vi "XML Build Entity.vi"(0 "Attributes":string[](array[string]), 1 "level":i32, 3 "spaces per level":i32, 5 "Entity Name":string, 7 "Is Array?":bool, 9 "Has Children":bool, 11 "error in (no error)":errorcluster, 12 "Child Entities":string[](array[string])) -> (6 "Entity XML":string, 15 "error out":errorcluster)   [LabVIEW 2016]
doc: "PBrooks - 29 Oct 2018\n\nAdded space to Close Entity? string suffix for compliance to XML spec"
uses:
  <userlib>/_OpenG.lib/array/array.llb/Filter 1D Array (String)__ogtk.vi
  <userlib>/_OpenG.lib/array/array.llb/Empty 1D Array (String)__ogtk.vi
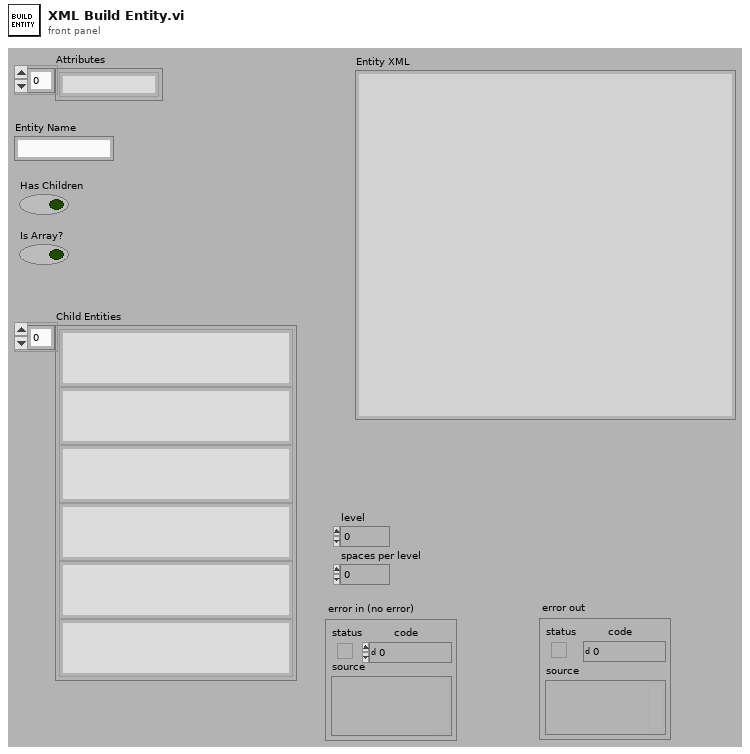
[diagram p1: front panel]
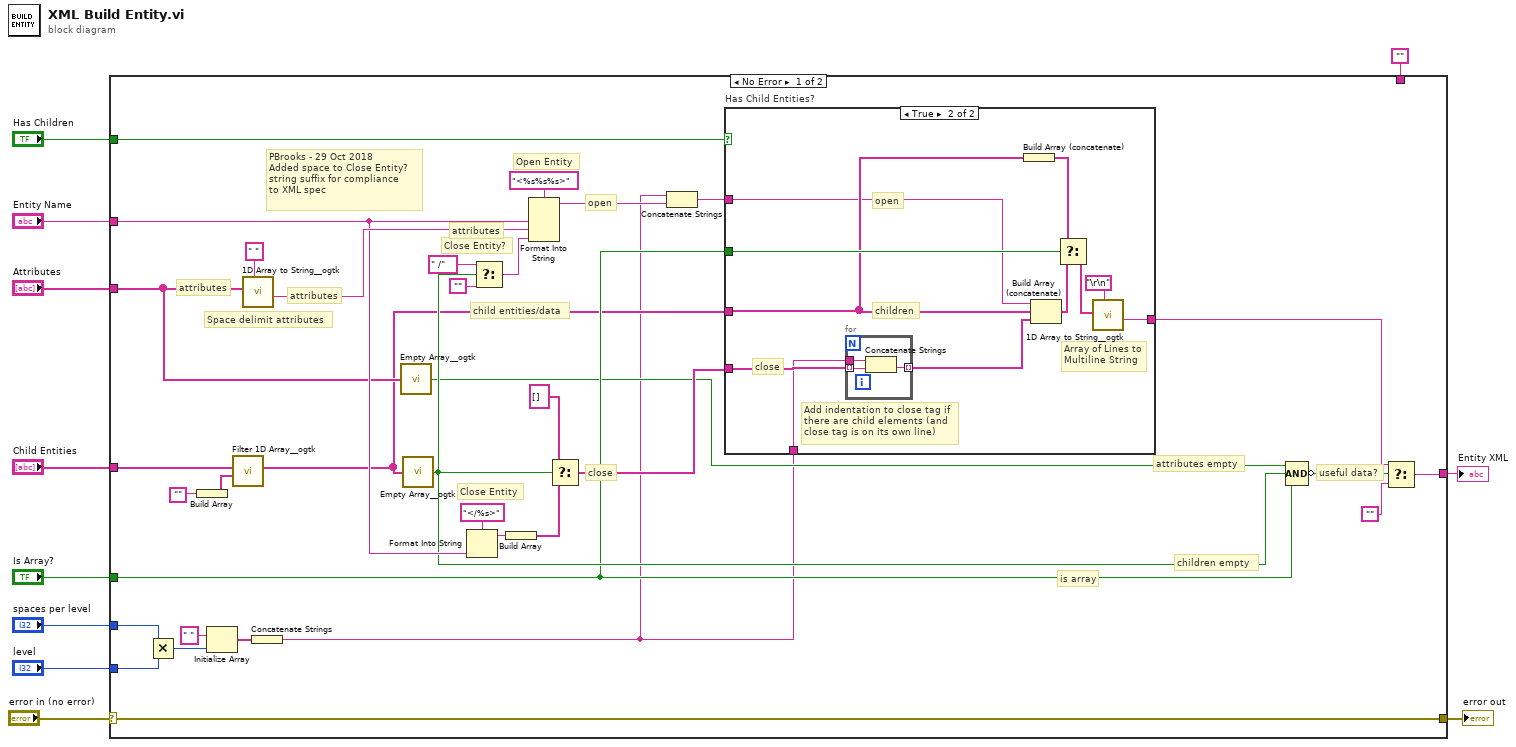
[diagram p0: block diagram]
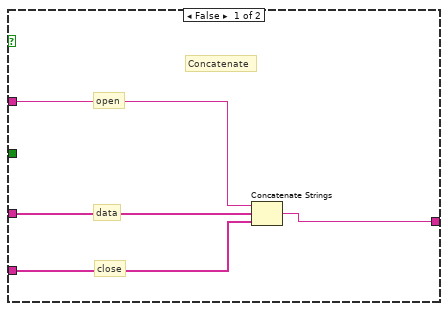
[diagram p2: hidden frame]
diagram:
  n1 = case shown="No Error" "error in (no error)" {
    selector: "error in (no error)" -> [w12 w65]
    tunnel: "Has Children" -> [w45 _]
    tunnel: "Entity Name" -> [w34 _]
    tunnel: "Attributes" -> [w32 _]
    tunnel: "Is Array?" -> [w30 _]
    tunnel: [w26 w64] -> w7
    tunnel: "Child Entities" -> [w23 _]
    tunnel: "spaces per level" -> [w19 _]
    tunnel: "level" -> [w18 _]
    tunnel: [w12 w65] -> w2
    tunnel: "" -> [_ w64]
    frame No Error {
      # "PBrooks - 29 Oct 2018\nAdded space to Close Entity?\nstring suffix for compliance\nto XML spec"
      # "useful data?"
      # "is array"
      # "children empty"
      # "attributes empty"
      # "attributes"
      # "open"
      # "close"
      # "child entities/data"
      # "attributes"
      # "attributes"
      # "Space delimit attributes"
      # "Close Entity?"
      # "Open Entity"
      # "Close Entity"
      n2 = Multiply(x=w19, y=w18) -> (x*y=w17:i32)
      n3 = Build Array("") -> (w21:string[])
      n4 = Initialize Array(" " ("delimiter (Tab)"), w17) -> (w20:string[])
      n5 = call-poly <userlib>:"Filter 1D Array__ogtk.vi"("items to filter"=w21, "array"=w23) -> ("filtered array"=w24:string[])  [unwired: 4 in, 1 out]
      n6 = call <userlib>:"1D Array to String__ogtk.vi"("delimiter (Tab)"=" ", "Array of Strings"=w32) -> ("delimited string"=w36:string)  [unwired: 9 in]
      n7 = Concatenate Strings(w20) -> (w13:string)
      n8 = call-poly <userlib>:"Empty Array__ogtk.vi"("Array"=w32) -> ("Empty Array?"=w25:bool)  [unwired: 8 in]
      n9 = call-poly <userlib>:"Empty Array__ogtk.vi"("Array"=w24) -> ("Empty Array?"=w31:bool)  [unwired: 8 in]
      n10 = Format Into String(format string="</%s>", w34) -> (resulting string=w38:string)  [unwired: 2 in, 1 out]
      n11 = Select(t=" /", s=w31, f="") -> (s? t:f=w41:string)
      n12 = Build Array(w38) -> (w43:string[])
      n13 = Format Into String(format string="<%s%s%s>", w34, w36, w41) -> (resulting string=w15:string)  [unwired: 2 in, 1 out]
      n14 = Select(t=string[] [], s=w31, f=w43) -> (s? t:f=w39:string[])
      n15 = Concatenate Strings(w13, w15) -> (w14:string)
      n16 = case "Has Child Entities?" shown="True" w45 {
        tunnel: w14 -> [w46 w50]
        tunnel: w39 -> [w47 w54]
        tunnel: [w48 w59] -> w28
        tunnel: w24 -> [w49 w51]
        tunnel: w30 -> [_ w58]
        tunnel: w13 -> [_ w52]
        frame False {
          # "close"
          # "open"
          # "data"
          # "Concatenate"
          n17 = Concatenate Strings(w46, w49, w47) -> (w48:string)
        }
        frame True {
          # "Add indentation to close tag if there are child elements (and close tag is on its own line)"
          # "close"
          # "open"
          # "children"
          # "Array of Lines to Multiline String"
          n18 = for {
            tunnel: w54 -> [w63] mode=indexing
            tunnel: [w61] -> w53 mode=indexing
            tunnel: w52 -> [w62]
            n19 = Concatenate Strings(w62, w63) -> (w61:string)
          }
          n20 = Build Array (concatenate)(w51) -> (w57:string[])
          n21 = Build Array (concatenate)(w50, w51, w53) -> (w56:string[])
          n22 = Select(t=w57, s=w58, f=w56) -> (s? t:f=w55:string[])
          n23 = call <userlib>:"1D Array to String__ogtk.vi"("delimiter (Tab)"="\r\n", "Array of Strings"=w55) -> ("delimited string"=w59:string)  [unwired: 9 in]
        }
      }
      n24 = Compound Arithmetic op=AND(w25, w31, w30) -> (invert w29:bool)
      n25 = Select(t=w28, s=w29, f="") -> (s? t:f=w26:string)
    }
    frame Error {
    }
  }
  "Entity XML" <- w7
  "error out" <- w2
